vi "SerialWrite.vi"(8 "error in (no error)":errorcluster, 10 "Text":string, 11 "VISA Refnum in":refnum<visa-resource-name>) -> (0 "error out":errorcluster, 3 "VISA Refnum out":refnum<visa-resource-name>)   [LabVIEW 2020]
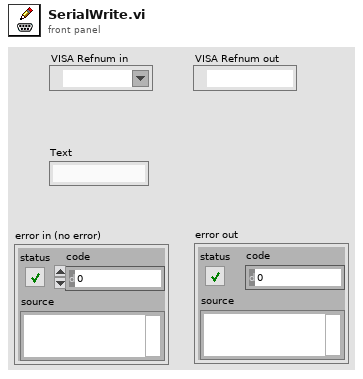
[diagram p1: front panel]
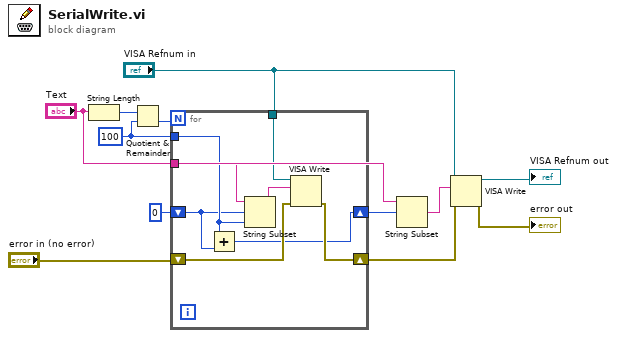
[diagram p0: block diagram]
diagram:
  w8 = 100 ("y")
  n1 = String Length(string="Text") -> (length=w12:i32)
  n2 = Quotient & Remainder(x=w12, y=w8) -> (floor(x/y)=w11:i32)  [unwired: 1 out]
  n3 = for {
    N: w11 -> [_]
    tunnel: "Text" -> [w17]
    tunnel: "VISA Refnum in" -> [w19]
    shift-right: [w18] -> w4
    shift-left: "error in (no error)" -> [w20]
    shift-right: [w14] -> w5
    shift-left: 0 ("y") -> [w15]
    tunnel: w8 -> [w16]
    n4 = Add(x=w16, y=w15) -> (x+y=w14:i32)
    n5 = String Subset(string=w17, offset (0)=w15, length (rest)=w16) -> (substring=w13:string)
    n6 = VISA Write(VISA resource name=w19, write buffer=w13, error in (no error)=w20) -> (error out=w18:errorcluster)  [unwired: 2 out]
  }
  n7 = String Subset(string="Text", offset (0)=w5) -> (substring=w6:string)  [unwired: 1 in]
  n8 = VISA Write(VISA resource name="VISA Refnum in", write buffer=w6, error in (no error)=w4) -> (VISA resource name out=→"VISA Refnum out":refnum<visa-resource-name>, error out=→"error out":errorcluster)  [unwired: 1 out]
